vi "set_PID.vi"(8 "error in (no error)":errorcluster, 10 "wavelength (nm)":string="632.99109", 11 "port":i32=2 min=1 max=2) -> (0 "error out":errorcluster, 2 "return type":i32)   [LabVIEW 2017, in "highfinesse.lvlib"]
uses:
  highfinesse.lvlib
  wlmData.dll
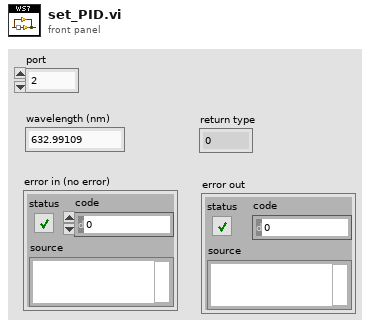
[diagram p1: front panel]
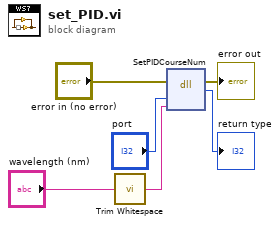
[diagram p0: block diagram]
diagram:
  n1 = call <vilib>:"Trim Whitespace.vi"("string"="wavelength (nm)") -> ("trimmed string"=w2:string)  [unwired: 1 in]
  n2 = dll-call lib="wlmData.dll" fn="SetPIDCourseNum"(error in="error in (no error)", "arg1"="port", "arg2"=w2) -> (error out=→"error out":errorcluster, "return type"=→"return type":i32)  [unwired: 4 in, 1 out]
